vi "Write Positions to Config.vi"(11 "Positions":dbl[](array[numeric])) -> (0 "error out":errorcluster)   [LabVIEW 2020, in "ESP301.lvlib"]
uses:
  ESP301.lvlib
  <vilib>/Utility/config.llb/Write Key (String).vi
  <vilib>/Utility/config.llb/NI_LVConfig.lvlib
panel:
  out "spreadsheet string":string
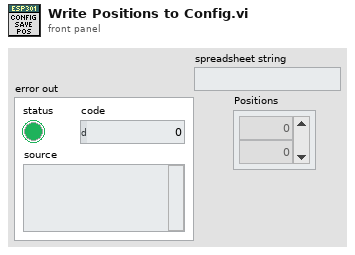
[diagram p1: front panel]
types:
  T1 = typedef "NI_LVConfig.lvlib/Config Data RefNum.ctl" = refnum<k1>
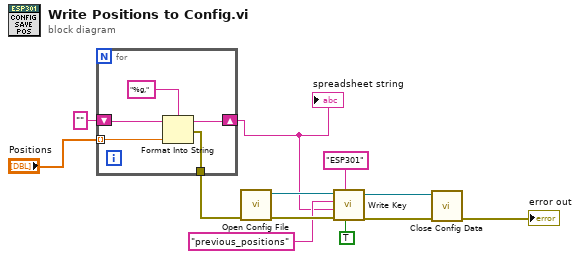
[diagram p0: block diagram]
diagram:
  n1 = for {
    tunnel: "Positions" -> [w17] mode=indexing
    shift-right: [w15] -> w2
    shift-left: "" -> [w16]
    tunnel: [w13] -> w3
    n2 = Format Into String(format string="%g,", initial string=w16, w17) -> (resulting string=w15:string, error out=w13:errorcluster)  [unwired: 1 in]
  }
  "spreadsheet string" <- w2
  n3 = call "Open Config File.vi"("error in (no error)"=w3) -> ("error out"=w12:errorcluster, "Refnum out"=w9:T1)  [unwired: 9 in]
  n4 = call-poly <vilib>:"Write Key.vi"("write raw string? (F)"=TRUE, "section"="ESP301", "error in (no error)"=w12, "value"=w2, "key"="previous_positions", "refnum"=w9) -> ("error out"=w11:errorcluster, "refnum out"=w6:T1)  [unwired: 3 in, 1 out]
  n5 = call <vilib>:"Close Config Data.vi"("error in (no error)"=w11, "refnum"=w6) -> ("error out"=→"error out":errorcluster)  [unwired: 8 in, 1 out]
